vi "findError.vi"(1 "error string in":string) -> (0 "error out":string)   [LabVIEW 2012, in "HGF_GPG.lvlib" / "HGF_GPG.lvclass"]
doc: "in error case this VI checks the returning string to read the error type"
uses:
  HGF_GPG.lvclass
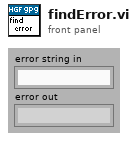
[diagram p1: front panel]
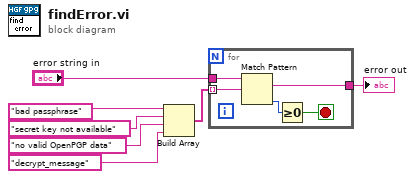
[diagram p0: block diagram]
diagram:
  n1 = Build Array("bad passphrase", "secret key not available", "no valid OpenPGP data", "decrypt_message") -> (w3:string[])
  n2 = for {
    tunnel: "error string in" -> [w12]
    tunnel: w3 -> [w11] mode=indexing
    tunnel: [w8] -> w2
    stop <- w9 stop-if-true
    n3 = Match Pattern(string=w12, regular expression=w11) -> (match substring=w8:string, offset past match=w10:i32)  [unwired: 3 out]
    n4 = Greater Or Equal To 0?(x=w10) -> (x >= 0?=w9:bool)
  }
  "error out" <- w2
